vi "example.vi"() -> ()   [LabVIEW 2013]
uses:
  LVAPI/dbm.lvclass
panel:
  out "Error out":errorcluster
  out "Value":string
  in  "Parameter":string="power"
  in  "ID":i32=1
  in  "Measurement":string="test_measurement"
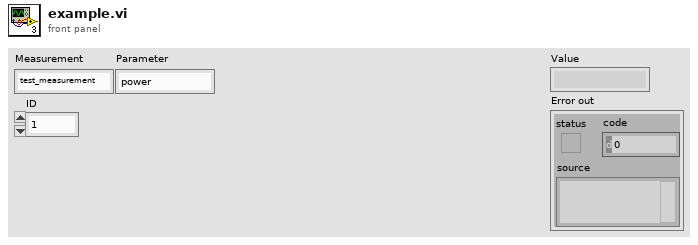
[diagram p1: front panel]
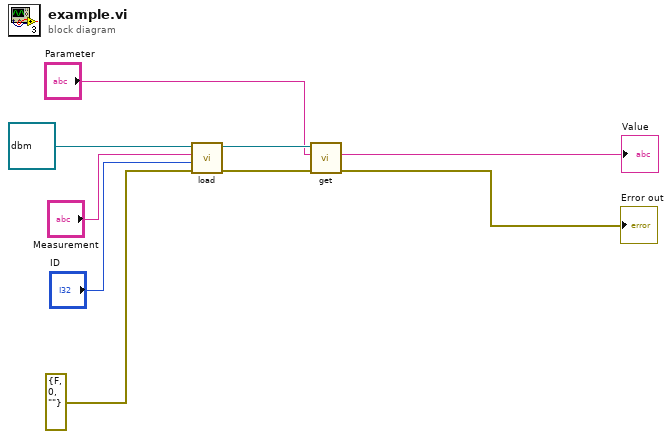
[diagram p0: block diagram]
diagram:
  n1 = call-dynamic "load.vi"("error in (no error)"=errorcluster {"status"=FALSE, "code"=0, "source"=""}, "ID"="ID", "Measurement"="Measurement", "dbm in"=refnum<class "dbm.lvclass"> refnum) -> ("error out"=w5:errorcluster, "dbm out"=w6:refnum<class "dbm.lvclass">)  [unwired: 6 in]
  n2 = call-dynamic "get.vi"("error in (no error)"=w5, "Parameter"="Parameter", "dbm in"=w6) -> ("error out"=→"Error out":errorcluster, "Value"=→"Value":string)  [unwired: 6 in, 1 out]
